vi "Add DataTable Variable (double).vi"(8 "error in (no error)":errorcluster, 9 "value":dbl, 10 "name":string, 11 "JMP DataTable":refnum<k7>) -> (0 "error out":errorcluster, 3 "JMP data table out":refnum<k7>)   [LabVIEW 2019, in "JMP Automation.lvlib"]
doc: "Add columns with their coresponding data to a DataDable"
uses:
  <instrlib>/LV_JMP_bridge/JMP Automation.lvlib
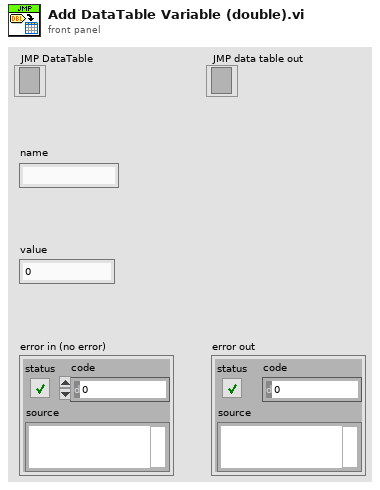
[diagram p1: front panel]
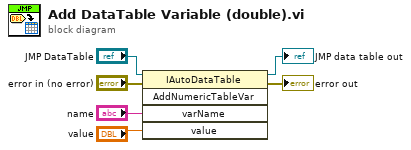
[diagram p0: block diagram]
diagram:
  n1 = invoke class="IAutoDataTable" method="AddNumericTableVar"(reference="JMP DataTable", error in="error in (no error)", "varName"="name", "value"="value") -> (reference out=→"JMP data table out":refnum<k7>, error out=→"error out":errorcluster)  [unwired: 1 in, 3 out]
